vi "Mode3.vi"() -> ()   [LabVIEW 2017]
uses:
  Classes/Sequence/SequenceSubvis/TestStep-StepType.ctl
  Classes/Sequence/SequenceSubvis/TestStepTypes.ctl
  Classes/Sequence/SequenceSubvis/RF Direction.ctl
  Classes/Sequence/SequenceSubvis/PolarizationSelect.ctl
  <vilib>/Utility/file.llb/Read Delimited Spreadsheet (DBL).vi
panel:
  in  "Antenna Tx/Rx":bool
  in  "H/V":bool
  out "PAARD Super Mode":T4(array[cluster])
  in  "PAARD Mode 1":T5[](array[typedef])
  in  "UCAR Super Sequence":T5[](array[typedef])
  # "Polarization = Probe Polarization"
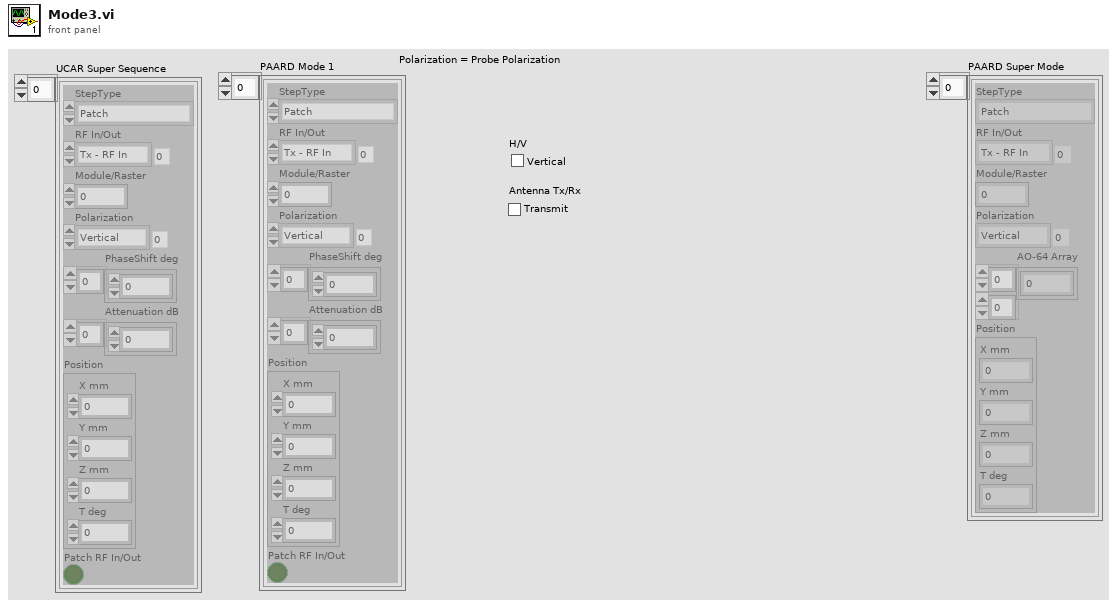
[diagram p1: front panel]
types:
  T1 = typedef "TestStepTypes.ctl" = enum16{"Patch", "Motion", "SweepTest", "RasterTest", "Finish", "64ModuleCfg"}
  T2 = typedef "RF Direction.ctl" = enum16{"Tx - RF In", "Rx - RF Out"}
  T3 = typedef "PolarizationSelect.ctl" = enum16{"Vertical", "Horizontal"}
  T4 = cluster{"StepType":T1, "RF In/Out":T2, "Module/Raster":i32, "Polarization":T3, "AO-64 Array":dbl[][], "Position":cluster{"X mm":dbl, "Y mm":dbl, "Z mm":dbl, "T deg":dbl}}[]
  T5 = typedef "TestStep-StepType.ctl" = cluster{"StepType":T1, "RF In/Out":T2, "Module/Raster":i32, "Polarization":T3, "PhaseShift deg":dbl[], "Attenuation dB":dbl[], "Position":cluster{"X mm":dbl, "Y mm":dbl, "Z mm":dbl, "T deg":dbl}, "Patch RF In/Out":bool}
  T6 = cluster{"StepType":T1, "RF In/Out":T2, "Module/Raster":i32, "Polarization":T3, "AO-64 Array":dbl[][], "Position":cluster{"X mm":dbl, "Y mm":dbl, "Z mm":dbl, "T deg":dbl}}
  T7 = cluster{"X mm":dbl, "Y mm":dbl, "File Path":path}[]
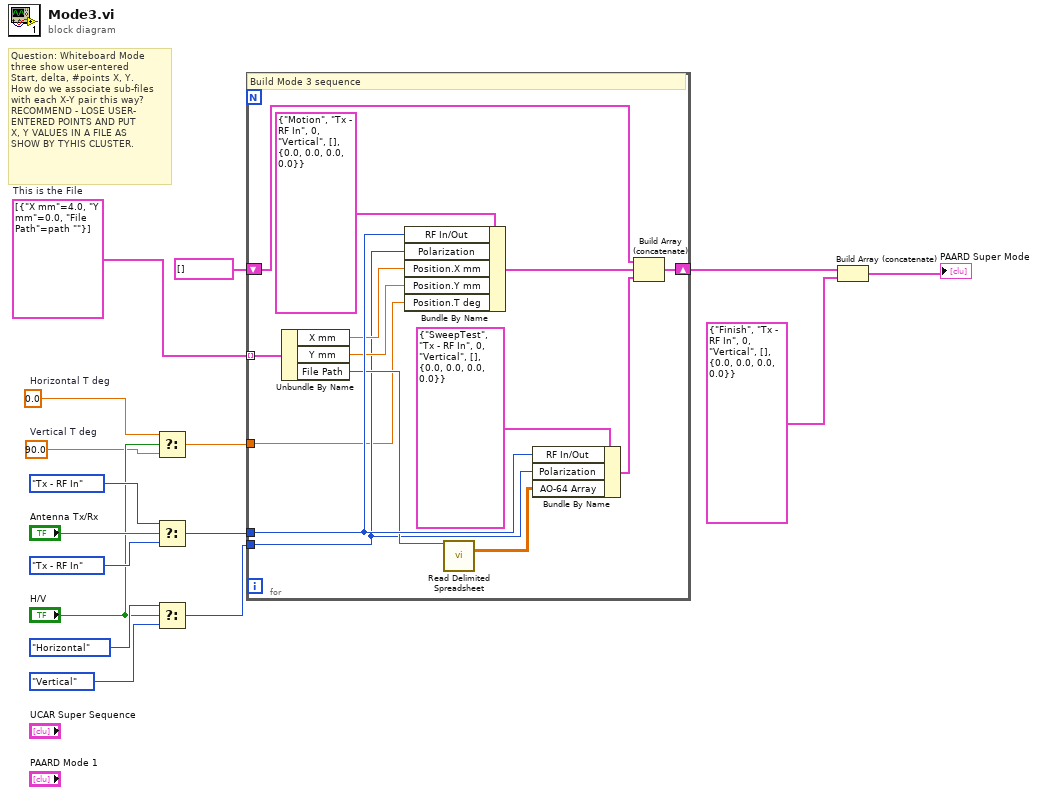
[diagram p0: block diagram]
diagram:
  w6 = 90.0  # Vertical T deg
  w7 = 0.0  # Horizontal T deg
  w9 = T7 [{"X mm"=4.0, "Y mm"=0.0, "File Path"=path ""}]  # This is the File
  # "Question: Whiteboard Mode\nthree show user-entered\nStart, delta, #points X, Y.\nHow do we associate sub-files\nwith each X-Y pair this way?\nRECOMMEND - LOSE USER-\nENTERED POINTS AND PUT \nX, Y VALUES IN A FILE AS\nSHOW BY TYHIS CLUSTER."
  n1 = Select(t=w7, s="H/V", f=w6) -> (s? t:f=w4:dbl)
  n2 = Select(t=RF_Direction."Tx - RF In" ("RF In/Out"), s="Antenna Tx/Rx", f=RF_Direction."Tx - RF In" ("RF In/Out")) -> (s? t:f=w11:T2)
  n3 = Select(t=PolarizationSelect."Horizontal" ("Polarization"), s="H/V", f=PolarizationSelect."Vertical" ("Polarization")) -> (s? t:f=w10:T3)
  n4 = for {
    tunnel: w11 -> [w28]
    tunnel: w10 -> [w20]
    tunnel: w9 -> [w27] mode=indexing
    shift-right: [w19] -> w3
    shift-left: T4 [] -> [w18]
    tunnel: w4 -> [w17]
    # "Build Mode 3 sequence"
    n5 = Unbundle By Name(w27) -> ("X mm"=w25:dbl, "Y mm"=w24:dbl, "File Path"=w26:path)
    n6 = Bundle By Name(cluster=T6 {"StepType"=enum."Motion", "RF In/Out"=enum."Tx - RF In", "Module/Raster"=0, "Polarization"=enum."Vertical", "AO-64 Array"=[], "Position"={"X mm"=0.0, "Y mm"=0.0, "Z mm"=0.0, "T deg"=0.0}} ("Test"), "RF In/Out"=w28, "Polarization"=w20, "Position.X mm"=w25, "Position.Y mm"=w24, "Position.T deg"=w17) -> (w22:T6)
    n7 = call-poly <vilib>:"Read Delimited Spreadsheet.vi"("file path (dialog if empty)"=w26) -> ("all rows"=w23:dbl[][])  [unwired: 9 in, 5 out]
    n8 = Bundle By Name(cluster=T6 {"StepType"=enum."SweepTest", "RF In/Out"=enum."Tx - RF In", "Module/Raster"=0, "Polarization"=enum."Vertical", "AO-64 Array"=[], "Position"={"X mm"=0.0, "Y mm"=0.0, "Z mm"=0.0, "T deg"=0.0}} ("Test"), "RF In/Out"=w28, "Polarization"=w20, "AO-64 Array"=w23) -> (w21:T6)
    n9 = Build Array (concatenate)(w18, w22, w21) -> (w19:T4)
  }
  n10 = Build Array (concatenate)(w3, T6 {"StepType"=enum."Finish", "RF In/Out"=enum."Tx - RF In", "Module/Raster"=0, "Polarization"=enum."Vertical", "AO-64 Array"=[], "Position"={"X mm"=0.0, "Y mm"=0.0, "Z mm"=0.0, "T deg"=0.0}} ("Test")) -> (→"PAARD Super Mode":T4)
